vi "ADITYA VENDING MACHINE.vi"() -> ()   [LabVIEW 2019]
uses:
  Control 1.ctl
panel:
  out "TEA":dbl(slide) scale=0.0..10.0
  out "COFFEE":dbl(slide) scale=0.0..10.0
  in  "MENU":T1
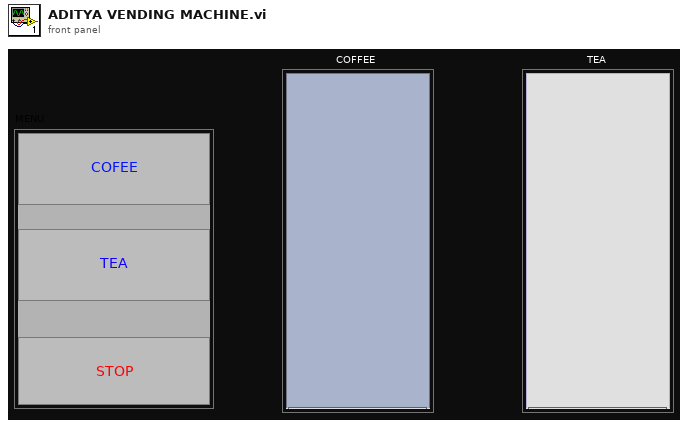
[diagram p1: front panel]
types:
  T1 = cluster{"CANCEL BUTTON":bool, " TEA":bool, "stop":bool}
  T2 = typedef "Control 1.ctl" = enum32{"Ideal", "Coffee", "Tea", "Stop"}
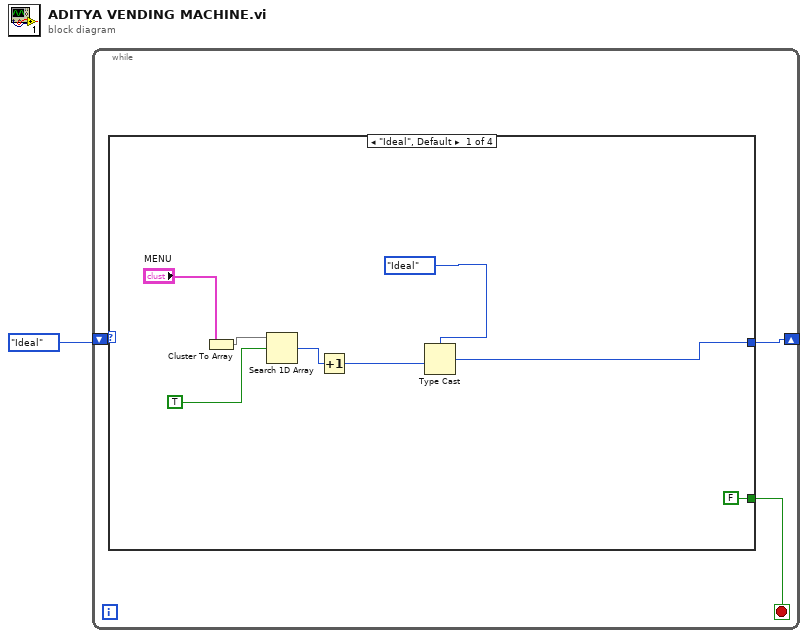
[diagram p0: block diagram]
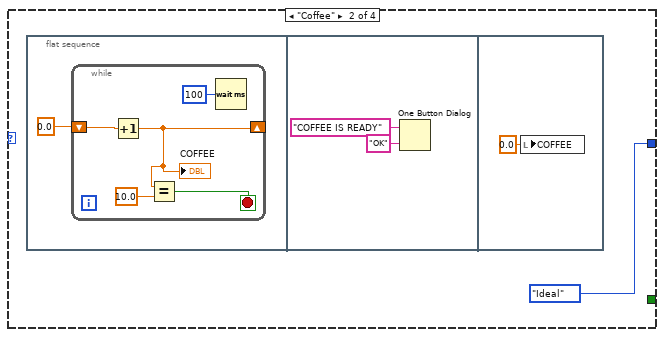
[diagram p2: hidden frame]
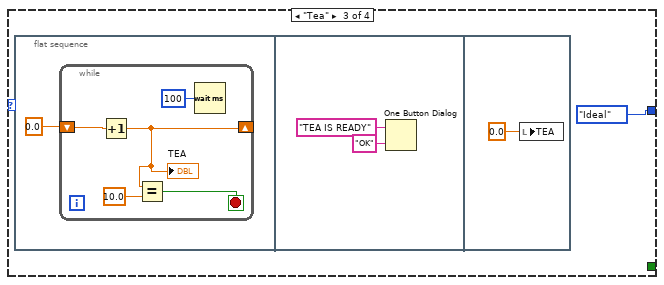
[diagram p3: hidden frame]
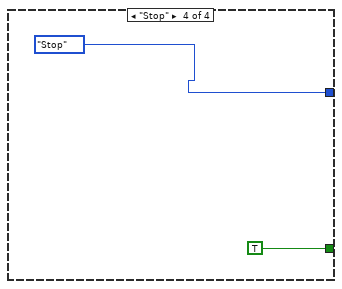
[diagram p4: hidden frame]
diagram:
  n1 = while {
    shift-right: [w3] -> _
    shift-left: Control_1."Ideal" -> [w4]
    stop <- w2 stop-if-true
    n2 = case shown="\"Ideal\", Default" w4 {
      tunnel: [w10 Control_1."Ideal" Control_1."Ideal" Control_1."Stop"] -> w3
      tunnel: [FALSE _ _ TRUE] -> w2
      frame "Ideal", Default {
        n3 = Cluster To Array(cluster="MENU") -> (array=w12:bool[])
        n4 = Search 1D Array(1D array=w12, element=TRUE) -> (index of element=w11:i32)  [unwired: 1 in]
        n5 = Increment(x=w11) -> (x+1=w7:i32)
        n6 = Type Cast(type=Control_1."Ideal", x=w7) -> (*(type *) &x=w10:T2)
      }
      frame "Coffee" {
        n7 = flat-sequence {
          frame #0 {
            n8 = while {
              shift-right: [w18] -> _
              shift-left: 0.0 -> [w19]
              stop <- w16 stop-if-true
              n9 = Increment(x=w19) -> (x+1=w18:dbl)
              "COFFEE" <- w18
              n10 = Equal?(x=w18, y=10.0) -> (x = y?=w16:bool)
              n11 = Wait (ms)(milliseconds to wait=u32 100) -> ()  [unwired: 1 out]
            }
          }
          frame #1 {
            n12 = One Button Dialog(message="COFFEE IS READY", button name ("OK")="OK") -> ()  [unwired: 1 out]
          }
          frame #2 {
            n13 = local write "COFFEE"(0.0 ("COFFEE")) -> ()
          }
        }
      }
      frame "Tea" {
        n14 = flat-sequence {
          frame #0 {
            n15 = while {
              shift-right: [w28] -> _
              shift-left: 0.0 -> [w29]
              stop <- w26 stop-if-true
              n16 = Increment(x=w29) -> (x+1=w28:dbl)
              "TEA" <- w28
              n17 = Equal?(x=w28, y=10.0) -> (x = y?=w26:bool)
              n18 = Wait (ms)(milliseconds to wait=u32 100) -> ()  [unwired: 1 out]
            }
          }
          frame #1 {
            n19 = One Button Dialog(message="TEA IS READY", button name ("OK")="OK") -> ()  [unwired: 1 out]
          }
          frame #2 {
            n20 = local write "TEA"(0.0 ("COFFEE")) -> ()
          }
        }
      }
      frame "Stop" {
      }
    }
  }
